vi "상태머신.vi"() -> ()   [LabVIEW 2014]
uses:
  Status.ctl
  <vilib>/Analysis/NI_AALBase.lvlib
panel:
  out "웨이브폼 그래프":dbl[](graph)
  in  "사인파 생성":bool
  in  "정지":bool
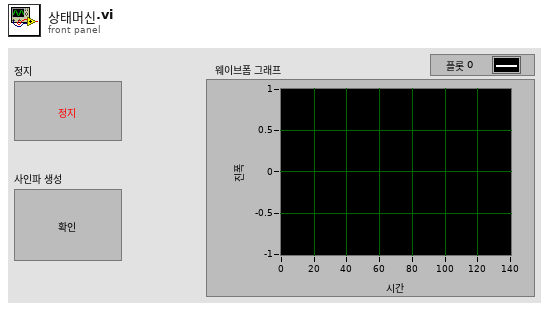
[diagram p1: front panel]
types:
  T1 = typedef "Status.ctl" = enum16{"Idle", "초기화", "정지", "Task1", "Task2", "기다림"}
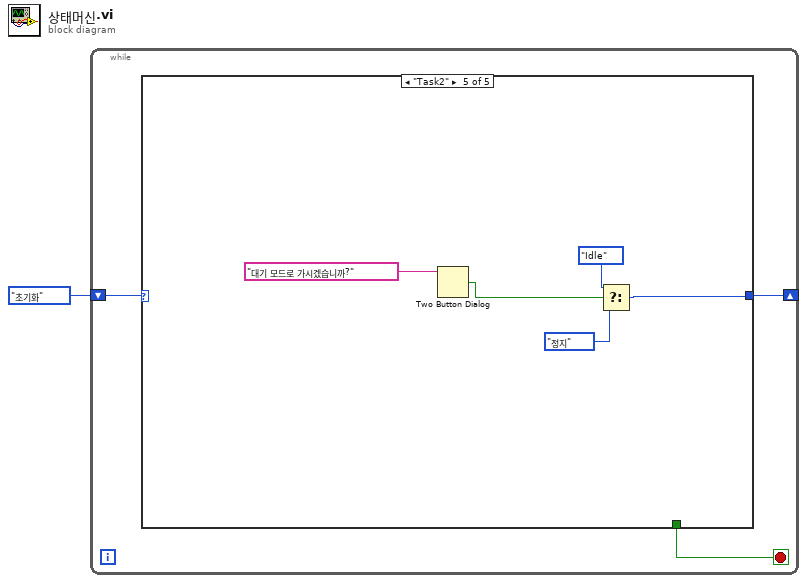
[diagram p0: block diagram]
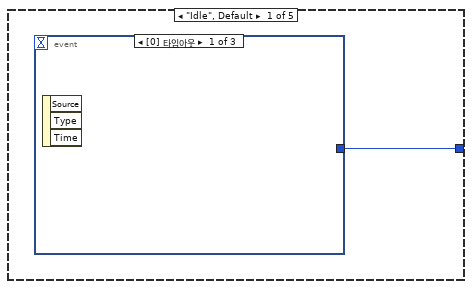
[diagram p2: hidden frame]
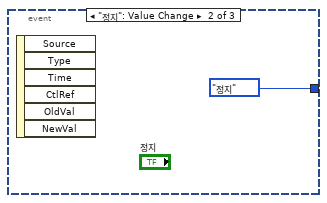
[diagram p3: hidden frame]
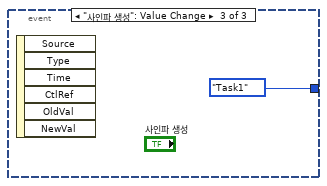
[diagram p4: hidden frame]
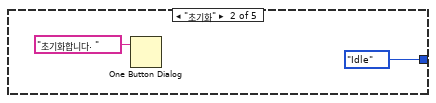
[diagram p5: hidden frame]
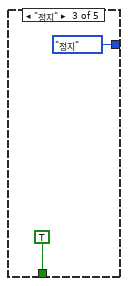
[diagram p6: hidden frame]
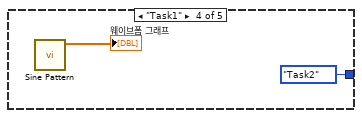
[diagram p7: hidden frame]
diagram:
  n1 = while {
    shift-right: [w3] -> _
    shift-left: Status."초기화" ("상태") -> [w4]
    stop <- w2 stop-if-true
    n2 = case shown="\"Task2\"" w4 {
      tunnel: [w5 Status."Idle" ("상태") Status."정지" ("상태") Status."Task2" ("상태") w14] -> w3
      tunnel: [_ _ TRUE _ _] -> w2
      frame "Idle", Default {
        n3 = event shown="[0] 타임아웃" {
          selector: _ -> [_ _ _]
          dyn-events: _ -> [_ _ _]
          timeout: _ -> [_ _ _]
          tunnel: [_ Status."정지" ("상태") Status."Task1" ("상태")] -> w5
          event Timeout {
            n4 = event-data() -> ()  [unwired: 1 in, 3 out]
          }
          event "정지": Value Change {
            n5 = event-data() -> ()  [unwired: 1 in, 6 out]
          }
          event "사인파 생성": Value Change {
            n6 = event-data() -> ()  [unwired: 1 in, 6 out]
          }
        }
      }
      frame "초기화" {
        n7 = One Button Dialog(message="초기화합니다. " ("메시지")) -> ()  [unwired: 1 in, 1 out]
      }
      frame "정지" {
      }
      frame "Task1" {
        n8 = call <vilib>:"Sine Pattern.vi"() -> ("Sinusoidal Pattern"=→"웨이브폼 그래프":dbl[])  [unwired: 4 in, 1 out]
      }
      frame "Task2" {
        n9 = Two Button Dialog(message="대기 모드로 가시겠습니까?" ("메시지")) -> (T button?=w17:bool)  [unwired: 2 in]
        n10 = Select(t=Status."Idle" ("상태"), s=w17, f=Status."정지" ("상태")) -> (s? t:f=w14:T1)
      }
    }
  }
